vi "AI Channel Filter.vi"(7 "Device Ref":T1 format="%.0x", 8 "error in (no error)":errorcluster caption="错误输入（无错误）", 11 "DIChannel":T2[](array[typedef])) -> (0 "error out":errorcluster caption="错误输出", 3 "DIChannel":T2[](array[typedef]))   [LabVIEW 2013]
uses:
  <vilib>/K2Labs/HiLab API/Custom Device API/Custom Device API Library.lvlib
  <vilib>/K2Labs/HiLab API/Custom Device API/Configuration/Item Properties/Get Item Property/Get Item Property(U32).vi
  <vilib>/K2Labs/HiLab API/Custom Device API/Configuration/Item Properties/Get Item Property/Get Item Property(String).vi
  <vilib>/Utility/miscctls.llb/LVRowAndColumnTypeDef.ctl
  AI Param.ctl
  <vilib>/K2Labs/HiLab API/Custom Device API/Controls/Custom Device Item Reference.ctl
panel:
  in  "Lists":i32[](listbox) caption="通道与信号的对应关系筛查列表"
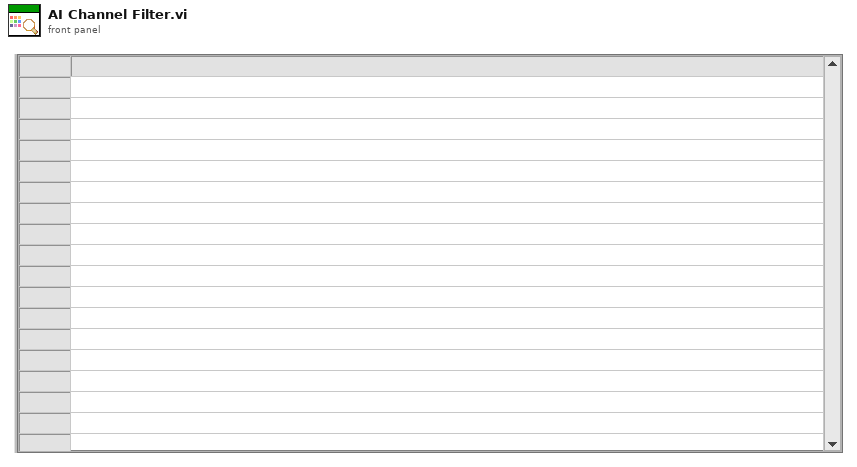
[diagram p1: front panel]
types:
  T1 = typedef "Custom Device API Library.lvlib/Custom Device Item Reference.ctl" = u64
  T2 = typedef "AI Param.ctl" = cluster{"Name":string, "Description":string, "DefaultValue":dbl, "Physical Channel":string}
  T3 = typedef "LVRowAndColumnTypeDef.ctl" = cluster{"Row":i32, "Column":i32}
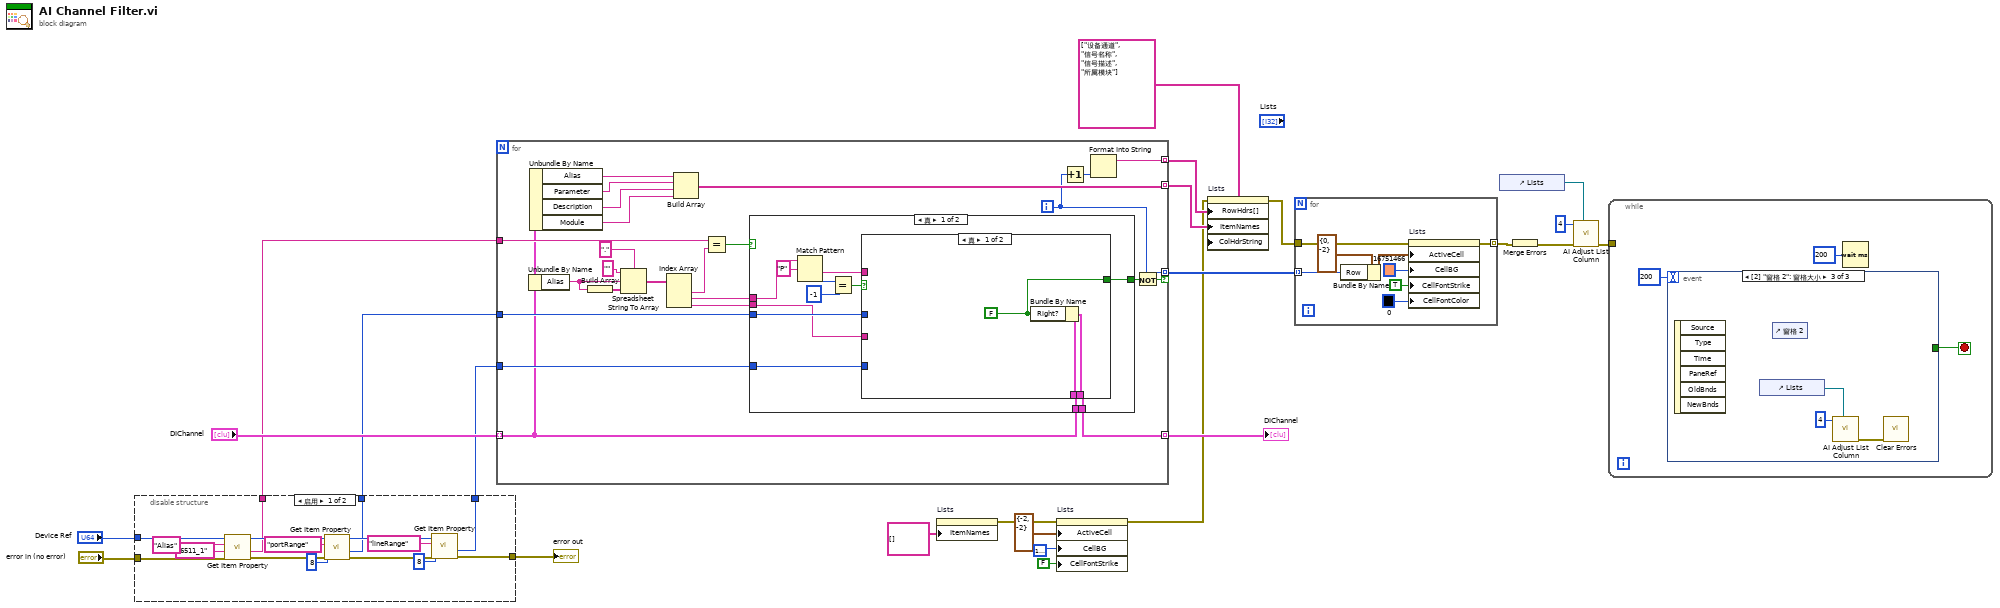
[diagram p0: block diagram]
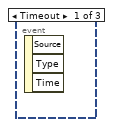
[diagram p2: hidden frame]
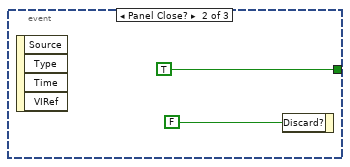
[diagram p3: hidden frame]
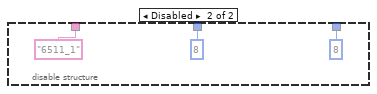
[diagram p4: hidden frame]
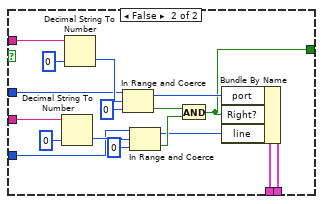
[diagram p5: hidden frame]
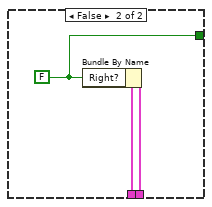
[diagram p6: hidden frame]
diagram:
  n1 = disable-structure shown="启用" {
    disable-tunnel: "Device Ref" -> [w40 _]
    disable-tunnel: [w25 "6511_1" ("Value")] -> w22
    disable-tunnel: [w32 u32 8 ("Value")] -> w21
    disable-tunnel: [w31 u32 8 ("Value")] -> w20
    disable-tunnel: [w27 _] -> w19
    disable-tunnel: "error in (no error)" -> [w26 _]
    frame Enabled {
      n2 = call-poly <vilib>:"Get Item Property.vi"("error in (no error)"=w26, "Default Value"="6511_1", "Property Name"="Alias", "Item Ref in"=w40) -> ("error out"=w37:errorcluster, "Value"=w25:string, "Item Ref out"=w38:T1)  [unwired: 4 in, 1 out]
      n3 = call-poly <vilib>:"Get Item Property.vi"("error in (no error)"=w37, "Default Value"=u32 8, "Property Name"="portRange", "Item Ref in"=w38) -> ("error out"=w34:errorcluster, "Value"=w32:u32, "Item Ref out"=w35:T1)  [unwired: 4 in, 1 out]
      n4 = call-poly <vilib>:"Get Item Property.vi"("error in (no error)"=w34, "Default Value"=u32 8, "Property Name"="lineRange", "Item Ref in"=w35) -> ("error out"=w27:errorcluster, "Value"=w31:u32)  [unwired: 4 in, 2 out]
    }
    frame Disabled {
    }
  }
  "error out" <- w19
  n5 = for {
    tunnel: "DIChannel" -> [w54] mode=indexing
    tunnel: [w67] -> w17 mode=indexing
    tunnel: w22 -> [w62]
    tunnel: w21 -> [w56]
    tunnel: w20 -> [w55]
    tunnel: [w49] -> w9 mode=indexing
    tunnel: [w46] -> w15 mode=indexing if=w47
    tunnel: [w44] -> w8 mode=indexing
    i -> [w46]
    n6 = Unbundle By Name(w54) -> ("Alias"=w57:string)
    n7 = Unbundle By Name(w54) -> ("Alias"=w53:string, "Parameter"=w52:string, "Description"=w51:string, "Module"=w50:string)
    n8 = Build Array(w57) -> (w66:string[])
    n9 = Spreadsheet String To Array(delimiter (Tab)="." ("分隔符(Tab)"), format string="" ("格式字符串"), spreadsheet string=w57, array type (2D Dbl)=w66) -> (array=w63:string[])
    n10 = Index Array(array=w63) -> (element #1=w60:string, element #2=w59:string, element #3=w58:string)  [unwired: 3 in]
    n11 = Build Array(w53, w52, w51, w50) -> (w49:string[])
    n12 = Equal?(x=w62, y=w60) -> (x = y?=w61:bool)
    n13 = case shown="真" w61 {
      tunnel: [w79 w102] -> w67
      tunnel: w54 -> [w78 w101]
      tunnel: w59 -> [w77 _]
      tunnel: w58 -> [w70 _]
      tunnel: w56 -> [w71 _]
      tunnel: w55 -> [w69 _]
      tunnel: [w68 w100] -> w48
      frame True {
        n14 = Match Pattern(string=w77, regular expression="P" ("正则表达式")) -> (after substring=w72:string, offset past match=w75:i32)  [unwired: 1 in, 2 out]
        n15 = Equal?(x=w75, y=-1) -> (x = y?=w73:bool)
        n16 = case shown="真" w73 {
          tunnel: [w82 w99] -> w79
          tunnel: w78 -> [w81 w98]
          tunnel: w72 -> [_ w97]
          tunnel: w71 -> [_ w95]
          tunnel: w70 -> [_ w88]
          tunnel: w69 -> [_ w87]
          tunnel: [w80 w83] -> w68
          frame True {
            w80 = FALSE ("Right?")
            n17 = Bundle By Name(cluster=w81, "Right?"=w80) -> (w82:T2)
          }
          frame False {
            n18 = Decimal String To Number(string=w88, default (0L)=u32 0 ("默认(0 I32)")) -> (number=w91:u32)  [unwired: 1 in, 1 out]
            n19 = Decimal String To Number(string=w97, default (0L)=u32 0 ("默认(0 I32)")) -> (number=w96:u32)  [unwired: 1 in, 1 out]
            n20 = In Range and Coerce(upper limit=w95, x=w96, lower limit=u32 0 ("下限")) -> (coerced(x)=w92:u32, In Range?=w86:bool)
            n21 = In Range and Coerce(upper limit=w87, x=w91, lower limit=u32 0 ("下限")) -> (coerced(x)=w84:u32, In Range?=w85:bool)
            n22 = And(x=w86, y=w85) -> (x .and. y?=w83:bool)
            n23 = Bundle By Name(cluster=w98, "port"=w92, "Right?"=w83, "line"=w84) -> (w99:T2)
          }
        }
      }
      frame False {
        w100 = FALSE ("Right?")
        n24 = Bundle By Name(cluster=w101, "Right?"=w100) -> (w102:T2)
      }
    }
    n25 = Increment(x=w46) -> (x+1=w45:i32)
    n26 = Format Into String(w45) -> (resulting string=w44:string)  [unwired: 3 in, 1 out]
    n27 = Not(x=w48) -> (.not. x?=w47:bool)
  }
  "DIChannel" <- w17
  n28 = property on="Lists" class="MCListbox (严格)"("ItemNames"=string[][] [] ("项名")) -> (error out=w6:errorcluster)  [unwired: 2 in, 1 out]
  n29 = property on="Lists" class="MCListbox (严格)"(error in=w6, "ActiveCell"=T3 {"Row"=-2, "Column"=-2} ("活动单元格:活动单元格"), "CellBG"=u32 16777225, "CellFontStrike"=FALSE ("活动单元格:单元格字体:删除线")) -> (error out=w5:errorcluster)  [unwired: 1 in, 1 out]
  n30 = property on="Lists" class="MCListbox (严格)"(error in=w5, "RowHdrs[]"=w8, "ItemNames"=w9, "ColHdrString"=string[] ["设备通道", "信号名称", "信号描述", "所属模块"] ("列首字符串[]")) -> (error out=w16:errorcluster)  [unwired: 1 in, 1 out]
  n31 = for {
    tunnel: w16 -> [w110]
    tunnel: w15 -> [w107] mode=indexing
    tunnel: [w103] -> w14 mode=indexing
    n32 = Bundle By Name(cluster=T3 {"Row"=0, "Column"=-2} ("活动单元格:活动单元格"), "Row"=w107) -> (w108:T3)
    n33 = property on="Lists" class="MCListbox (严格)"(error in=w110, "ActiveCell"=w108, "CellBG"=u32 16751466, "CellFontStrike"=TRUE ("活动单元格:单元格字体:删除线"), "CellFontColor"=u32 0) -> (error out=w103:errorcluster)  [unwired: 1 in, 1 out]
  }
  n34 = control-ref of="Lists"() -> (w13:refnum<vi>)
  n35 = Merge Errors(w14) -> (w11:errorcluster)
  n36 = call "AI Adjust List Column.vi"("List"=w13, "error in (no error)"=w11, "Column"=4) -> ("error out"=w10:errorcluster)  [unwired: 8 in]
  n37 = while {
    tunnel: w10 -> [_]
    stop <- w112 stop-if-true
    n38 = event shown="[2] \"窗格 2\": 窗格大小" {
      selector: _ -> [_ _ _]
      dyn-events: _ -> [_ _ _]
      timeout: 200 -> [_ _ _]
      tunnel: [_ TRUE _] -> w112
      event Timeout {
        n39 = event-data() -> ()  [unwired: 1 in, 3 out]
      }
      event Panel Close? {
        n40 = event-data() -> ()  [unwired: 1 in, 4 out]
        n41 = event-data("Discard?"=FALSE ("放弃？")) -> ()  [unwired: 1 in, 1 out]
      }
      event Pane Size {
        n42 = event-data() -> ()  [unwired: 1 in, 6 out]
        n43 = control-ref of="Lists"() -> (w117:refnum<vi>)
        n44 = control-ref of="窗格 2"() -> ()  [unwired: 1 out]
        n45 = call "AI Adjust List Column.vi"("List"=w117, "Column"=4) -> ("error out"=w116:errorcluster)  [unwired: 9 in]
        n46 = call <vilib>:"Clear Errors.vi"("error in (no error)"=w116) -> ()  [unwired: 6 in, 1 out]
      }
    }
    n47 = Wait (ms)(milliseconds to wait=u32 200 ("等待时间（毫秒）")) -> ()  [unwired: 1 out]
  }
